vi "Generate LO Reconfiguration.vi"(0 "rx configs":T3(array[cluster]), 5 "coerced configs":T4(array[cluster])) -> (4 "lo configs":T1(array[cluster]))   [LabVIEW 2021]
uses:
  Start Trigger.ctl
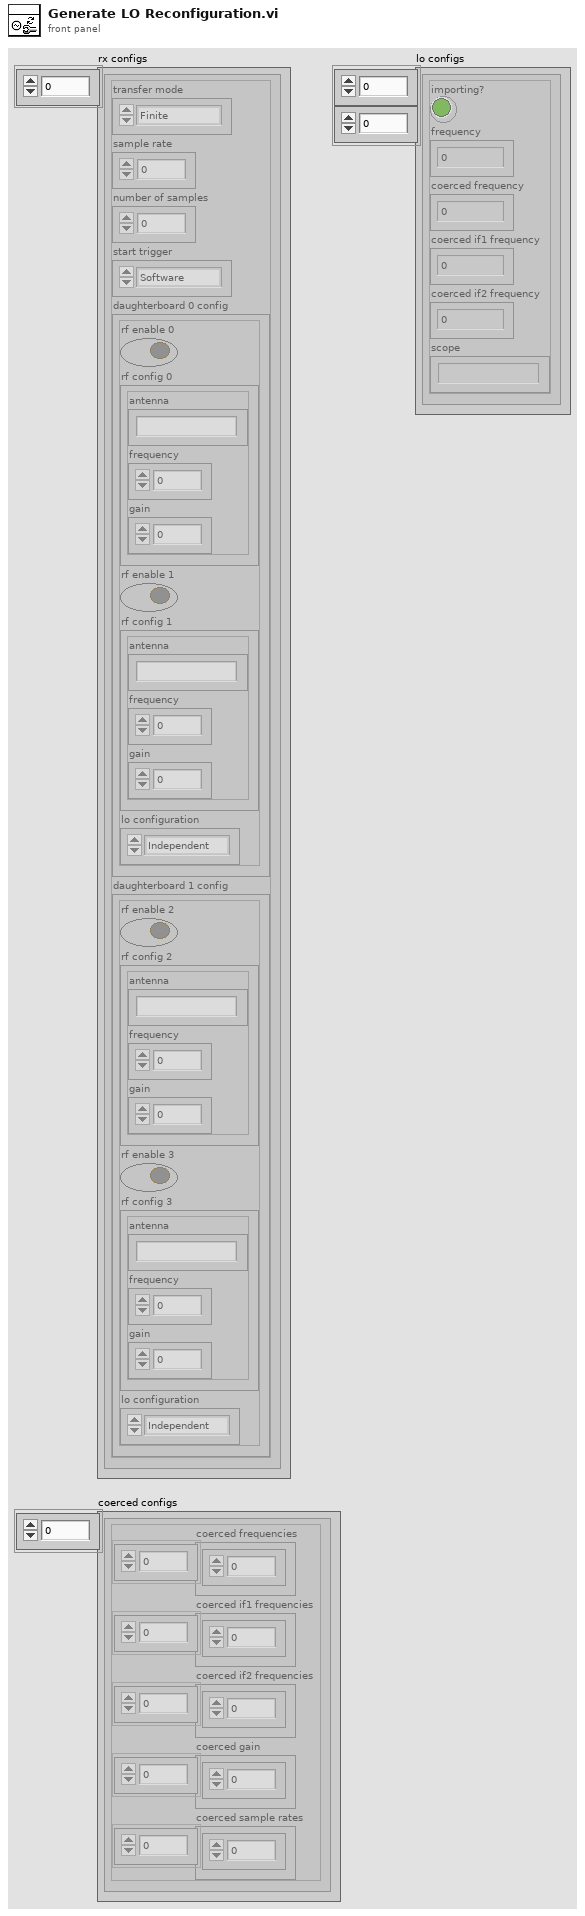
[diagram p1: front panel]
types:
  T1 = cluster{"importing?":bool, "frequency":dbl, "coerced frequency":dbl, "coerced if1 frequency":dbl, "coerced if2 frequency":dbl, "scope":string}[][]
  T2 = typedef "Start Trigger.ctl" = enum8{"Software", "Digital Edge", "Rx Start Trigger", "Tx Start Trigger", "Immediate", "Future Time Event"}
  T3 = cluster{"transfer mode":enum16{"Finite", "Continuous"}, "sample rate":dbl, "number of samples":u32, "start trigger":T2, "daughterboard 0 config":cluster{"rf enable 0":bool, "rf config 0":cluster{"antenna":string, "frequency":dbl, "gain":dbl}, "rf enable 1":bool, "rf config 1":cluster{"antenna":string, "frequency":dbl, "gain":dbl}, "lo configuration":enum16{"Independent", "Import", "Shared and Export", "Reimport", "Shared"}}, "daughterboard 1 config":cluster{"rf enable 2":bool, "rf config 2":cluster{"antenna":string, "frequency":dbl, "gain":dbl}, "rf enable 3":bool, "rf config 3":cluster{"antenna":string, "frequency":dbl, "gain":dbl}, "lo configuration":enum16{"Independent", "Import", "Shared and Export", "Reimport", "Shared"}}}[]
  T4 = cluster{"coerced frequencies":dbl[], "coerced if1 frequencies":dbl[], "coerced if2 frequencies":dbl[], "coerced gain":dbl[], "coerced sample rates":dbl[]}[]
  T5 = cluster{"importing?":bool, "frequency":dbl, "coerced frequency":dbl, "coerced if1 frequency":dbl, "coerced if2 frequency":dbl, "scope":string}
  T6 = enum16{"Independent", "Import", "Shared and Export", "Reimport", "Shared"}
  T7 = enum16{"Independent", "Import", "Shared and Export", "Reimport", "Shared"}[]
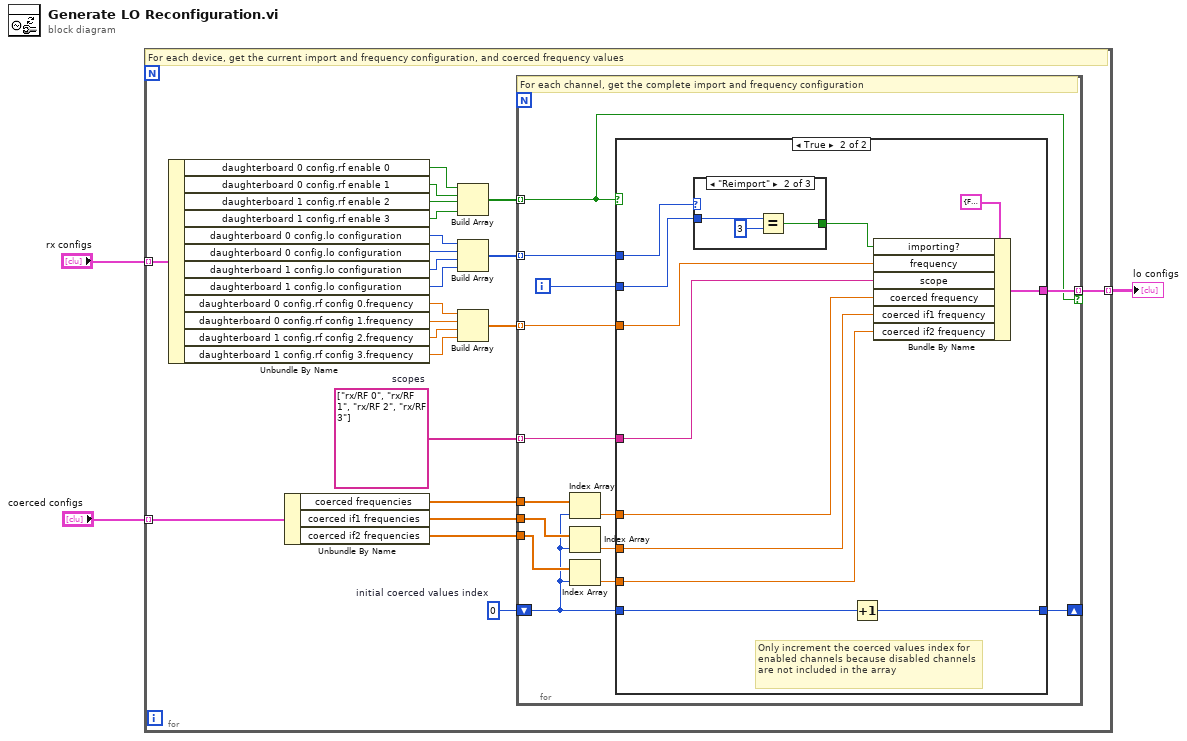
[diagram p0: block diagram]
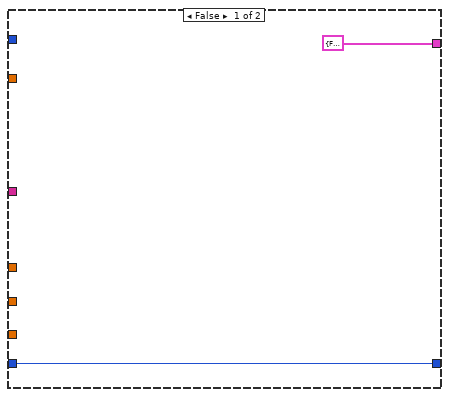
[diagram p2: hidden frame]
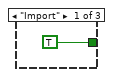
[diagram p3: hidden frame]
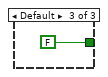
[diagram p4: hidden frame]
diagram:
  n1 = for {
    tunnel: "rx configs" -> [w26] mode=indexing
    tunnel: "coerced configs" -> [w16] mode=indexing
    tunnel: [w5] -> w1 mode=indexing
    w6 = string[] ["rx/RF 0", "rx/RF 1", "rx/RF 2", "rx/RF 3"]  # scopes
    w12 = 0  # initial coerced values index
    # "For each device, get the current import and frequency configuration, and coerced frequency values"
    n2 = Unbundle By Name(w26) -> ("daughterboard 0 config.rf enable 0"=w25:bool, "daughterboard 0 config.rf enable 1"=w24:bool, "daughterboard 1 config.rf enable 2"=w23:bool, "daughterboard 1 config.rf enable 3"=w4:bool, "daughterboard 0 config.lo configuration"=w22:T6, "daughterboard 0 config.lo configuration"=w21:T6, "daughterboard 1 config.lo configuration"=w20:T6, "daughterboard 1 config.lo configuration"=w19:T6, "daughterboard 0 config.rf config 0.frequency"=w10:dbl, "daughterboard 0 config.rf config 1.frequency"=w9:dbl, "daughterboard 1 config.rf config 2.frequency"=w11:dbl, "daughterboard 1 config.rf config 3.frequency"=w8:dbl)
    n3 = Unbundle By Name(w16) -> ("coerced frequencies"=w15:dbl[], "coerced if1 frequencies"=w13:dbl[], "coerced if2 frequencies"=w14:dbl[])
    n4 = Build Array(w25, w24, w23, w4) -> (w18:bool[])
    n5 = Build Array(w22, w21, w20, w19) -> (w17:T7)
    n6 = Build Array(w10, w9, w11, w8) -> (w7:dbl[])
    n7 = for {
      tunnel: w18 -> [w28] mode=indexing
      tunnel: w17 -> [w34] mode=indexing
      tunnel: w15 -> [w38]
      tunnel: w14 -> [w39]
      tunnel: w13 -> [w40]
      shift-right: [w31] -> _
      shift-left: w12 -> [w33]
      tunnel: w7 -> [w32] mode=indexing
      tunnel: w6 -> [w30] mode=indexing
      tunnel: [w29] -> w5 mode=indexing if=w28
      i -> [w27]
      # "For each channel, get the complete import and frequency configuration"
      n8 = Index Array(array=w38, index=w33) -> (element=w35:dbl)
      n9 = Index Array(array=w40, index=w33) -> (element=w36:dbl)
      n10 = Index Array(array=w39, index=w33) -> (element=w37:dbl)
      n11 = case shown="True" w28 {
        tunnel: w33 -> [w41 w50]
        tunnel: w37 -> [_ w53]
        tunnel: w36 -> [_ w52]
        tunnel: w35 -> [_ w48]
        tunnel: w34 -> [_ w45]
        tunnel: w32 -> [_ w51]
        tunnel: [w41 w49] -> w31
        tunnel: w30 -> [_ w47]
        tunnel: [T5 {"importing?"=FALSE, "frequency"=0.0, "coerced frequency"=0.0, "coerced if1 frequency"=0.0, "coerced if2 frequency"=0.0, "scope"=""} w46] -> w29
        tunnel: w27 -> [_ w43]
        frame False {
        }
        frame True {
          # "Only increment the coerced values index for enabled channels because disabled channels are not included in the array"
          n12 = case shown="\"Reimport\"" w45 {
            tunnel: [TRUE w56 FALSE] -> w44
            tunnel: w43 -> [_ w58 _]
            frame "Import" {
            }
            frame "Reimport" {
              n13 = Equal?(x=w58, y=3) -> (x = y?=w56:bool)
            }
            frame Default {
            }
          }
          n14 = Increment(x=w50) -> (x+1=w49:i32)
          n15 = Bundle By Name(cluster=T5 {"importing?"=FALSE, "frequency"=0.0, "coerced frequency"=0.0, "coerced if1 frequency"=0.0, "coerced if2 frequency"=0.0, "scope"=""}, "importing?"=w44, "frequency"=w51, "scope"=w47, "coerced frequency"=w48, "coerced if1 frequency"=w52, "coerced if2 frequency"=w53) -> (w46:T5)
        }
      }
    }
  }
  "lo configs" <- w1
